vi "lalalala.vi"() -> ()   [LabVIEW 2014]
uses:
  C:/Program Files (x86)/National Instruments/LabVIEW 2014/instr.lib/IDS/ueye.NET/uEyeDotNet.dll
  <vilib>/Analysis/NI_AALBase.lvlib
panel:
  out "Set 2":i32(ring) items=["SUCCESS, Success"=0, "IO_REQUEST_FAILED"=2, "CANT_OPEN_DEVICE"=3, "CANT_CLOSE_DEVICE"=4, "CANT_SETUP_MEMORY"=5, "NO_HWND_FOR_ERROR_REPORT"=6, "ERROR_MESSAGE_NOT_CREATED"=7, "ERROR_STRING_NOT_FOUND"=8, "HOOK_NOT_CREATED"=9, "TIMER_NOT_CREATED"=10, "CANT_OPEN_REGISTRY"=11, "CANT_READ_REGISTRY"=12, "CANT_VALIDATE_BOARD"=13, "CANT_GIVE_BOARD_ACCESS"=14, "NO_IMAGE_MEM_ALLOCATED"=15, "CANT_CLEANUP_MEMORY"=16, "CANT_COMMUNICATE_WITH_DRIVER"=17, "FUNCTION_NOT_SUPPORTED_YET"=18, "OPERATING_SYSTEM_NOT_SUPPORTED"=19, "INVALID_VIDEO_IN"=20, "INVALID_IMG_SIZE"=21, "INVALID_ADDRESS"=22, "INVALID_VIDEO_MODE"=23, "INVALID_AGC_MODE"=24, "INVALID_GAMMA_MODE"=25, "INVALID_SYNC_LEVEL"=26, "INVALID_CBARS_MODE"=27, "INVALID_COLOR_MODE"=28, "INVALID_SCALE_FACTOR"=29, "INVALID_IMAGE_SIZE"=30, "INVALID_IMAGE_POS"=31, "INVALID_CAPTURE_MODE"=32, "INVALID_RISC_PROGRAM"=33, "INVALID_BRIGHTNESS"=34, "INVALID_CONTRAST"=35, "INVALID_SATURATION_U"=36, "INVALID_SATURATION_V"=37, "INVALID_HUE"=38, "INVALID_HOR_FILTER_STEP"=39, "INVALID_VERT_FILTER_STEP"=40, "INVALID_EEPROM_READ_ADDRESS"=41, "INVALID_EEPROM_WRITE_ADDRESS"=42, "INVALID_EEPROM_READ_LENGTH"=43, "INVALID_EEPROM_WRITE_LENGTH"=44, "INVALID_BOARD_INFO_POINTER"=45, "INVALID_DISPLAY_MODE"=46, "INVALID_ERR_REP_MODE"=47, "INVALID_BITS_PIXEL"=48, "INVALID_MEMORY_POINTER"=49, "FILE_WRITE_OPEN_ERROR"=50, "FILE_READ_OPEN_ERROR"=51, "FILE_READ_INVALID_BMP_ID"=52, "FILE_READ_INVALID_BMP_SIZE"=53, "FILE_READ_INVALID_BIT_COUNT"=54, "WRONG_KERNEL_VERSION"=55, "RISC_INVALID_XLENGTH"=60, "RISC_INVALID_YLENGTH"=61, "RISC_EXCEED_IMG_SIZE"=62, "DD_MAIN_FAILED"=70, "DD_PRIMSURFACE_FAILED"=71, "DD_SCRN_SIZE_NOT_SUPPORTED"=72, "DD_CLIPPER_FAILED"=73, "DD_CLIPPER_HWND_FAILED"=74, "DD_CLIPPER_CONNECT_FAILED"=75, "DD_BACKSURFACE_FAILED"=76, "DD_BACKSURFACE_IN_SYSMEM"=77, "DD_MDL_MALLOC_ERR"=78, "DD_MDL_SIZE_ERR"=79, "DD_CLIP_NO_CHANGE"=80, "DD_PRIMMEM_NULL"=81, "DD_BACKMEM_NULL"=82, "DD_BACKOVLMEM_NULL"=83, "DD_OVERLAYSURFACE_FAILED"=84, "DD_OVERLAYSURFACE_IN_SYSMEM"=85, "DD_OVERLAY_NOT_ALLOWED"=86, "DD_OVERLAY_COLKEY_ERR"=87, "DD_OVERLAY_NOT_ENABLED"=88, "DD_GET_DC_ERROR"=89, "DD_DDRAW_DLL_NOT_LOADED"=90, "DD_THREAD_NOT_CREATED"=91, "DD_CANT_GET_CAPS"=92, "DD_NO_OVERLAYSURFACE"=93, "DD_NO_OVERLAYSTRETCH"=94, "DD_CANT_CREATE_OVERLAYSURFACE"=95, "DD_CANT_UPDATE_OVERLAYSURFACE"=96, "DD_INVALID_STRETCH"=97, "EV_INVALID_EVENT_NUMBER"=100, "INVALID_MODE"=101, "CANT_FIND_FALCHOOK, CANT_FIND_HOOK"=102, "CANT_GET_HOOK_PROC_ADDR"=103, "CANT_CHAIN_HOOK_PROC"=104, "CANT_SETUP_WND_PROC"=105, "HWND_NULL"=106, "INVALID_UPDATE_MODE"=107, "NO_ACTIVE_IMG_MEM"=108, "CANT_INIT_EVENT"=109, "FUNC_NOT_AVAIL_IN_OS"=110, "CAMERA_NOT_CONNECTED"=111, "SEQUENCE_LIST_EMPTY"=112, "CANT_ADD_TO_SEQUENCE"=113, "LOW_OF_SEQUENCE_RISC_MEM"=114, "IMGMEM2FREE_USED_IN_SEQ"=115, "IMGMEM_NOT_IN_SEQUENCE_LIST"=116, "SEQUENCE_BUF_ALREADY_LOCKED"=117, "INVALID_DEVICE_ID"=118, "INVALID_BOARD_ID"=119, "ALL_DEVICES_BUSY"=120, "HOOK_BUSY"=121, "TIMED_OUT"=122, "NULL_POINTER"=123, "WRONG_HOOK_VERSION"=124, "InvalidParameter, INVALID_PARAMETER"=125, "NOT_ALLOWED"=126, "OUT_OF_MEMORY"=127, "INVALID_WHILE_LIVE"=128, "ACCESS_VIOLATION"=129, "UNKNOWN_ROP_EFFECT"=130, "INVALID_RENDER_MODE"=131, "INVALID_THREAD_CONTEXT"=132, "NO_HARDWARE_INSTALLED"=133, "INVALID_WATCHDOG_TIME"=134, "INVALID_WATCHDOG_MODE"=135, "INVALID_PASSTHROUGH_IN"=136, "ERROR_SETTING_PASSTHROUGH_IN"=137, "FAILURE_ON_SETTING_WATCHDOG"=138, "NO_USB20"=139, "CAPTURE_RUNNING"=140, "MEMORY_BOARD_ACTIVATED"=141, "MEMORY_BOARD_DEACTIVATED"=142, "NO_MEMORY_BOARD_CONNECTED"=143, "TOO_LESS_MEMORY"=144, "IMAGE_NOT_PRESENT"=145, "MEMORY_MODE_RUNNING"=146, "MEMORYBOARD_DISABLED"=147, "TRIGGER_ACTIVATED"=148, "WRONG_KEY"=150, "CRC_ERROR"=151, "NOT_YET_RELEASED"=152, "NOT_CALIBRATED"=153, "WAITING_FOR_KERNEL"=154, "NOT_SUPPORTED"=155, "TRIGGER_NOT_ACTIVATED"=156, "OPERATION_ABORTED"=157, "BAD_STRUCTURE_SIZE"=158, "INVALID_BUFFER_SIZE"=159, "INVALID_PIXEL_CLOCK"=160, "INVALID_EXPOSURE_TIME"=161, "AUTO_EXPOSURE_RUNNING"=162, "CANNOT_CREATE_BB_SURF"=163, "CANNOT_CREATE_BB_MIX"=164, "BB_OVLMEM_NULL"=165, "CANNOT_CREATE_BB_OVL"=166, "NOT_SUPP_IN_OVL_SURF_MODE"=167, "INVALID_SURFACE"=168, "SURFACE_LOST"=169, "RELEASE_BB_OVL_DC"=170, "BB_TIMER_NOT_CREATED"=171, "BB_OVL_NOT_EN"=172, "ONLY_IN_BB_MODE"=173, "INVALID_COLOR_FORMAT"=174, "INVALID_WB_BINNING_MODE"=175, "INVALID_I2C_DEVICE_ADDRESS"=176, "COULD_NOT_CONVERT"=177, "TRANSFER_ERROR"=178, "PARAMETER_SET_NOT_PRESENT"=179, "INVALID_CAMERA_TYPE"=180, "INVALID_HOST_IP_HIBYTE"=181, "CM_NOT_SUPP_IN_CURR_DISPLAYMODE"=182, "NO_IR_FILTER"=183, "STARTER_FW_UPLOAD_NEEDED"=184, "LIBRARY_NOT_FOUND, DR_LIBRARY_NOT_FOUND"=185, "DR_DEVICE_OUT_OF_MEMORY, DEVICE_OUT_OF_MEMORY"=186, "DR_CANNOT_CREATE_SURFACE, CANNOT_CREATE_SURFACE"=187, "CANNOT_CREATE_VERTEX_BUFFER, DR_CANNOT_CREATE_VERTEX_BUFFER"=188, "CANNOT_CREATE_TEXTURE, DR_CANNOT_CREATE_TEXTURE"=189, "CANNOT_LOCK_OVERLAY_SURFACE, DR_CANNOT_LOCK_OVERLAY_SURFACE"=190, "DR_CANNOT_UNLOCK_OVERLAY_SURFACE, CANNOT_UNLOCK_OVERLAY_SURFACE"=191, "CANNOT_GET_OVERLAY_DC, DR_CANNOT_GET_OVERLAY_DC"=192, "DR_CANNOT_RELEASE_OVERLAY_DC, CANNOT_RELEASE_OVERLAY_DC"=193, "DEVICE_CAPS_INSUFFICIENT, DR_DEVICE_CAPS_INSUFFICIENT"=194, "INCOMPATIBLE_SETTING"=195, "DR_NOT_ALLOWED_WHILE_DC_IS_ACTIVE"=196, "DEVICE_ALREADY_PAIRED"=197, "SUBNETMASK_MISMATCH"=198, "SUBNET_MISMATCH"=199, "INVALID_IP_CONFIGURATION"=200, "DEVICE_NOT_COMPATIBLE"=201, "NETWORK_FRAME_SIZE_INCOMPATIBLE"=202, "NETWORK_CONFIGURATION_INVALID"=203, "ERROR_CPU_IDLE_STATES_CONFIGURATION"=204, "NoSuccess, NO_SUCCESS"=-1]
  out "s32Value":i32
  out "f64Value 2":dbl
  out "f64Value":dbl
  out "Set":i32(ring) items=["SUCCESS, Success"=0, "IO_REQUEST_FAILED"=2, "CANT_OPEN_DEVICE"=3, "CANT_CLOSE_DEVICE"=4, "CANT_SETUP_MEMORY"=5, "NO_HWND_FOR_ERROR_REPORT"=6, "ERROR_MESSAGE_NOT_CREATED"=7, "ERROR_STRING_NOT_FOUND"=8, "HOOK_NOT_CREATED"=9, "TIMER_NOT_CREATED"=10, "CANT_OPEN_REGISTRY"=11, "CANT_READ_REGISTRY"=12, "CANT_VALIDATE_BOARD"=13, "CANT_GIVE_BOARD_ACCESS"=14, "NO_IMAGE_MEM_ALLOCATED"=15, "CANT_CLEANUP_MEMORY"=16, "CANT_COMMUNICATE_WITH_DRIVER"=17, "FUNCTION_NOT_SUPPORTED_YET"=18, "OPERATING_SYSTEM_NOT_SUPPORTED"=19, "INVALID_VIDEO_IN"=20, "INVALID_IMG_SIZE"=21, "INVALID_ADDRESS"=22, "INVALID_VIDEO_MODE"=23, "INVALID_AGC_MODE"=24, "INVALID_GAMMA_MODE"=25, "INVALID_SYNC_LEVEL"=26, "INVALID_CBARS_MODE"=27, "INVALID_COLOR_MODE"=28, "INVALID_SCALE_FACTOR"=29, "INVALID_IMAGE_SIZE"=30, "INVALID_IMAGE_POS"=31, "INVALID_CAPTURE_MODE"=32, "INVALID_RISC_PROGRAM"=33, "INVALID_BRIGHTNESS"=34, "INVALID_CONTRAST"=35, "INVALID_SATURATION_U"=36, "INVALID_SATURATION_V"=37, "INVALID_HUE"=38, "INVALID_HOR_FILTER_STEP"=39, "INVALID_VERT_FILTER_STEP"=40, "INVALID_EEPROM_READ_ADDRESS"=41, "INVALID_EEPROM_WRITE_ADDRESS"=42, "INVALID_EEPROM_READ_LENGTH"=43, "INVALID_EEPROM_WRITE_LENGTH"=44, "INVALID_BOARD_INFO_POINTER"=45, "INVALID_DISPLAY_MODE"=46, "INVALID_ERR_REP_MODE"=47, "INVALID_BITS_PIXEL"=48, "INVALID_MEMORY_POINTER"=49, "FILE_WRITE_OPEN_ERROR"=50, "FILE_READ_OPEN_ERROR"=51, "FILE_READ_INVALID_BMP_ID"=52, "FILE_READ_INVALID_BMP_SIZE"=53, "FILE_READ_INVALID_BIT_COUNT"=54, "WRONG_KERNEL_VERSION"=55, "RISC_INVALID_XLENGTH"=60, "RISC_INVALID_YLENGTH"=61, "RISC_EXCEED_IMG_SIZE"=62, "DD_MAIN_FAILED"=70, "DD_PRIMSURFACE_FAILED"=71, "DD_SCRN_SIZE_NOT_SUPPORTED"=72, "DD_CLIPPER_FAILED"=73, "DD_CLIPPER_HWND_FAILED"=74, "DD_CLIPPER_CONNECT_FAILED"=75, "DD_BACKSURFACE_FAILED"=76, "DD_BACKSURFACE_IN_SYSMEM"=77, "DD_MDL_MALLOC_ERR"=78, "DD_MDL_SIZE_ERR"=79, "DD_CLIP_NO_CHANGE"=80, "DD_PRIMMEM_NULL"=81, "DD_BACKMEM_NULL"=82, "DD_BACKOVLMEM_NULL"=83, "DD_OVERLAYSURFACE_FAILED"=84, "DD_OVERLAYSURFACE_IN_SYSMEM"=85, "DD_OVERLAY_NOT_ALLOWED"=86, "DD_OVERLAY_COLKEY_ERR"=87, "DD_OVERLAY_NOT_ENABLED"=88, "DD_GET_DC_ERROR"=89, "DD_DDRAW_DLL_NOT_LOADED"=90, "DD_THREAD_NOT_CREATED"=91, "DD_CANT_GET_CAPS"=92, "DD_NO_OVERLAYSURFACE"=93, "DD_NO_OVERLAYSTRETCH"=94, "DD_CANT_CREATE_OVERLAYSURFACE"=95, "DD_CANT_UPDATE_OVERLAYSURFACE"=96, "DD_INVALID_STRETCH"=97, "EV_INVALID_EVENT_NUMBER"=100, "INVALID_MODE"=101, "CANT_FIND_FALCHOOK, CANT_FIND_HOOK"=102, "CANT_GET_HOOK_PROC_ADDR"=103, "CANT_CHAIN_HOOK_PROC"=104, "CANT_SETUP_WND_PROC"=105, "HWND_NULL"=106, "INVALID_UPDATE_MODE"=107, "NO_ACTIVE_IMG_MEM"=108, "CANT_INIT_EVENT"=109, "FUNC_NOT_AVAIL_IN_OS"=110, "CAMERA_NOT_CONNECTED"=111, "SEQUENCE_LIST_EMPTY"=112, "CANT_ADD_TO_SEQUENCE"=113, "LOW_OF_SEQUENCE_RISC_MEM"=114, "IMGMEM2FREE_USED_IN_SEQ"=115, "IMGMEM_NOT_IN_SEQUENCE_LIST"=116, "SEQUENCE_BUF_ALREADY_LOCKED"=117, "INVALID_DEVICE_ID"=118, "INVALID_BOARD_ID"=119, "ALL_DEVICES_BUSY"=120, "HOOK_BUSY"=121, "TIMED_OUT"=122, "NULL_POINTER"=123, "WRONG_HOOK_VERSION"=124, "InvalidParameter, INVALID_PARAMETER"=125, "NOT_ALLOWED"=126, "OUT_OF_MEMORY"=127, "INVALID_WHILE_LIVE"=128, "ACCESS_VIOLATION"=129, "UNKNOWN_ROP_EFFECT"=130, "INVALID_RENDER_MODE"=131, "INVALID_THREAD_CONTEXT"=132, "NO_HARDWARE_INSTALLED"=133, "INVALID_WATCHDOG_TIME"=134, "INVALID_WATCHDOG_MODE"=135, "INVALID_PASSTHROUGH_IN"=136, "ERROR_SETTING_PASSTHROUGH_IN"=137, "FAILURE_ON_SETTING_WATCHDOG"=138, "NO_USB20"=139, "CAPTURE_RUNNING"=140, "MEMORY_BOARD_ACTIVATED"=141, "MEMORY_BOARD_DEACTIVATED"=142, "NO_MEMORY_BOARD_CONNECTED"=143, "TOO_LESS_MEMORY"=144, "IMAGE_NOT_PRESENT"=145, "MEMORY_MODE_RUNNING"=146, "MEMORYBOARD_DISABLED"=147, "TRIGGER_ACTIVATED"=148, "WRONG_KEY"=150, "CRC_ERROR"=151, "NOT_YET_RELEASED"=152, "NOT_CALIBRATED"=153, "WAITING_FOR_KERNEL"=154, "NOT_SUPPORTED"=155, "TRIGGER_NOT_ACTIVATED"=156, "OPERATION_ABORTED"=157, "BAD_STRUCTURE_SIZE"=158, "INVALID_BUFFER_SIZE"=159, "INVALID_PIXEL_CLOCK"=160, "INVALID_EXPOSURE_TIME"=161, "AUTO_EXPOSURE_RUNNING"=162, "CANNOT_CREATE_BB_SURF"=163, "CANNOT_CREATE_BB_MIX"=164, "BB_OVLMEM_NULL"=165, "CANNOT_CREATE_BB_OVL"=166, "NOT_SUPP_IN_OVL_SURF_MODE"=167, "INVALID_SURFACE"=168, "SURFACE_LOST"=169, "RELEASE_BB_OVL_DC"=170, "BB_TIMER_NOT_CREATED"=171, "BB_OVL_NOT_EN"=172, "ONLY_IN_BB_MODE"=173, "INVALID_COLOR_FORMAT"=174, "INVALID_WB_BINNING_MODE"=175, "INVALID_I2C_DEVICE_ADDRESS"=176, "COULD_NOT_CONVERT"=177, "TRANSFER_ERROR"=178, "PARAMETER_SET_NOT_PRESENT"=179, "INVALID_CAMERA_TYPE"=180, "INVALID_HOST_IP_HIBYTE"=181, "CM_NOT_SUPP_IN_CURR_DISPLAYMODE"=182, "NO_IR_FILTER"=183, "STARTER_FW_UPLOAD_NEEDED"=184, "LIBRARY_NOT_FOUND, DR_LIBRARY_NOT_FOUND"=185, "DR_DEVICE_OUT_OF_MEMORY, DEVICE_OUT_OF_MEMORY"=186, "DR_CANNOT_CREATE_SURFACE, CANNOT_CREATE_SURFACE"=187, "CANNOT_CREATE_VERTEX_BUFFER, DR_CANNOT_CREATE_VERTEX_BUFFER"=188, "CANNOT_CREATE_TEXTURE, DR_CANNOT_CREATE_TEXTURE"=189, "CANNOT_LOCK_OVERLAY_SURFACE, DR_CANNOT_LOCK_OVERLAY_SURFACE"=190, "DR_CANNOT_UNLOCK_OVERLAY_SURFACE, CANNOT_UNLOCK_OVERLAY_SURFACE"=191, "CANNOT_GET_OVERLAY_DC, DR_CANNOT_GET_OVERLAY_DC"=192, "DR_CANNOT_RELEASE_OVERLAY_DC, CANNOT_RELEASE_OVERLAY_DC"=193, "DEVICE_CAPS_INSUFFICIENT, DR_DEVICE_CAPS_INSUFFICIENT"=194, "INCOMPATIBLE_SETTING"=195, "DR_NOT_ALLOWED_WHILE_DC_IS_ACTIVE"=196, "DEVICE_ALREADY_PAIRED"=197, "SUBNETMASK_MISMATCH"=198, "SUBNET_MISMATCH"=199, "INVALID_IP_CONFIGURATION"=200, "DEVICE_NOT_COMPATIBLE"=201, "NETWORK_FRAME_SIZE_INCOMPATIBLE"=202, "NETWORK_CONFIGURATION_INVALID"=203, "ERROR_CPU_IDLE_STATES_CONFIGURATION"=204, "NoSuccess, NO_SUCCESS"=-1]
  out "x/y":dbl
  out "Histogram Graph":T1(graph)
  out "Image":picture
  out "u8Image":u8[](array[numeric])
  out "CopyToArray":i32(ring) items=["SUCCESS, Success"=0, "IO_REQUEST_FAILED"=2, "CANT_OPEN_DEVICE"=3, "CANT_CLOSE_DEVICE"=4, "CANT_SETUP_MEMORY"=5, "NO_HWND_FOR_ERROR_REPORT"=6, "ERROR_MESSAGE_NOT_CREATED"=7, "ERROR_STRING_NOT_FOUND"=8, "HOOK_NOT_CREATED"=9, "TIMER_NOT_CREATED"=10, "CANT_OPEN_REGISTRY"=11, "CANT_READ_REGISTRY"=12, "CANT_VALIDATE_BOARD"=13, "CANT_GIVE_BOARD_ACCESS"=14, "NO_IMAGE_MEM_ALLOCATED"=15, "CANT_CLEANUP_MEMORY"=16, "CANT_COMMUNICATE_WITH_DRIVER"=17, "FUNCTION_NOT_SUPPORTED_YET"=18, "OPERATING_SYSTEM_NOT_SUPPORTED"=19, "INVALID_VIDEO_IN"=20, "INVALID_IMG_SIZE"=21, "INVALID_ADDRESS"=22, "INVALID_VIDEO_MODE"=23, "INVALID_AGC_MODE"=24, "INVALID_GAMMA_MODE"=25, "INVALID_SYNC_LEVEL"=26, "INVALID_CBARS_MODE"=27, "INVALID_COLOR_MODE"=28, "INVALID_SCALE_FACTOR"=29, "INVALID_IMAGE_SIZE"=30, "INVALID_IMAGE_POS"=31, "INVALID_CAPTURE_MODE"=32, "INVALID_RISC_PROGRAM"=33, "INVALID_BRIGHTNESS"=34, "INVALID_CONTRAST"=35, "INVALID_SATURATION_U"=36, "INVALID_SATURATION_V"=37, "INVALID_HUE"=38, "INVALID_HOR_FILTER_STEP"=39, "INVALID_VERT_FILTER_STEP"=40, "INVALID_EEPROM_READ_ADDRESS"=41, "INVALID_EEPROM_WRITE_ADDRESS"=42, "INVALID_EEPROM_READ_LENGTH"=43, "INVALID_EEPROM_WRITE_LENGTH"=44, "INVALID_BOARD_INFO_POINTER"=45, "INVALID_DISPLAY_MODE"=46, "INVALID_ERR_REP_MODE"=47, "INVALID_BITS_PIXEL"=48, "INVALID_MEMORY_POINTER"=49, "FILE_WRITE_OPEN_ERROR"=50, "FILE_READ_OPEN_ERROR"=51, "FILE_READ_INVALID_BMP_ID"=52, "FILE_READ_INVALID_BMP_SIZE"=53, "FILE_READ_INVALID_BIT_COUNT"=54, "WRONG_KERNEL_VERSION"=55, "RISC_INVALID_XLENGTH"=60, "RISC_INVALID_YLENGTH"=61, "RISC_EXCEED_IMG_SIZE"=62, "DD_MAIN_FAILED"=70, "DD_PRIMSURFACE_FAILED"=71, "DD_SCRN_SIZE_NOT_SUPPORTED"=72, "DD_CLIPPER_FAILED"=73, "DD_CLIPPER_HWND_FAILED"=74, "DD_CLIPPER_CONNECT_FAILED"=75, "DD_BACKSURFACE_FAILED"=76, "DD_BACKSURFACE_IN_SYSMEM"=77, "DD_MDL_MALLOC_ERR"=78, "DD_MDL_SIZE_ERR"=79, "DD_CLIP_NO_CHANGE"=80, "DD_PRIMMEM_NULL"=81, "DD_BACKMEM_NULL"=82, "DD_BACKOVLMEM_NULL"=83, "DD_OVERLAYSURFACE_FAILED"=84, "DD_OVERLAYSURFACE_IN_SYSMEM"=85, "DD_OVERLAY_NOT_ALLOWED"=86, "DD_OVERLAY_COLKEY_ERR"=87, "DD_OVERLAY_NOT_ENABLED"=88, "DD_GET_DC_ERROR"=89, "DD_DDRAW_DLL_NOT_LOADED"=90, "DD_THREAD_NOT_CREATED"=91, "DD_CANT_GET_CAPS"=92, "DD_NO_OVERLAYSURFACE"=93, "DD_NO_OVERLAYSTRETCH"=94, "DD_CANT_CREATE_OVERLAYSURFACE"=95, "DD_CANT_UPDATE_OVERLAYSURFACE"=96, "DD_INVALID_STRETCH"=97, "EV_INVALID_EVENT_NUMBER"=100, "INVALID_MODE"=101, "CANT_FIND_FALCHOOK, CANT_FIND_HOOK"=102, "CANT_GET_HOOK_PROC_ADDR"=103, "CANT_CHAIN_HOOK_PROC"=104, "CANT_SETUP_WND_PROC"=105, "HWND_NULL"=106, "INVALID_UPDATE_MODE"=107, "NO_ACTIVE_IMG_MEM"=108, "CANT_INIT_EVENT"=109, "FUNC_NOT_AVAIL_IN_OS"=110, "CAMERA_NOT_CONNECTED"=111, "SEQUENCE_LIST_EMPTY"=112, "CANT_ADD_TO_SEQUENCE"=113, "LOW_OF_SEQUENCE_RISC_MEM"=114, "IMGMEM2FREE_USED_IN_SEQ"=115, "IMGMEM_NOT_IN_SEQUENCE_LIST"=116, "SEQUENCE_BUF_ALREADY_LOCKED"=117, "INVALID_DEVICE_ID"=118, "INVALID_BOARD_ID"=119, "ALL_DEVICES_BUSY"=120, "HOOK_BUSY"=121, "TIMED_OUT"=122, "NULL_POINTER"=123, "WRONG_HOOK_VERSION"=124, "InvalidParameter, INVALID_PARAMETER"=125, "NOT_ALLOWED"=126, "OUT_OF_MEMORY"=127, "INVALID_WHILE_LIVE"=128, "ACCESS_VIOLATION"=129, "UNKNOWN_ROP_EFFECT"=130, "INVALID_RENDER_MODE"=131, "INVALID_THREAD_CONTEXT"=132, "NO_HARDWARE_INSTALLED"=133, "INVALID_WATCHDOG_TIME"=134, "INVALID_WATCHDOG_MODE"=135, "INVALID_PASSTHROUGH_IN"=136, "ERROR_SETTING_PASSTHROUGH_IN"=137, "FAILURE_ON_SETTING_WATCHDOG"=138, "NO_USB20"=139, "CAPTURE_RUNNING"=140, "MEMORY_BOARD_ACTIVATED"=141, "MEMORY_BOARD_DEACTIVATED"=142, "NO_MEMORY_BOARD_CONNECTED"=143, "TOO_LESS_MEMORY"=144, "IMAGE_NOT_PRESENT"=145, "MEMORY_MODE_RUNNING"=146, "MEMORYBOARD_DISABLED"=147, "TRIGGER_ACTIVATED"=148, "WRONG_KEY"=150, "CRC_ERROR"=151, "NOT_YET_RELEASED"=152, "NOT_CALIBRATED"=153, "WAITING_FOR_KERNEL"=154, "NOT_SUPPORTED"=155, "TRIGGER_NOT_ACTIVATED"=156, "OPERATION_ABORTED"=157, "BAD_STRUCTURE_SIZE"=158, "INVALID_BUFFER_SIZE"=159, "INVALID_PIXEL_CLOCK"=160, "INVALID_EXPOSURE_TIME"=161, "AUTO_EXPOSURE_RUNNING"=162, "CANNOT_CREATE_BB_SURF"=163, "CANNOT_CREATE_BB_MIX"=164, "BB_OVLMEM_NULL"=165, "CANNOT_CREATE_BB_OVL"=166, "NOT_SUPP_IN_OVL_SURF_MODE"=167, "INVALID_SURFACE"=168, "SURFACE_LOST"=169, "RELEASE_BB_OVL_DC"=170, "BB_TIMER_NOT_CREATED"=171, "BB_OVL_NOT_EN"=172, "ONLY_IN_BB_MODE"=173, "INVALID_COLOR_FORMAT"=174, "INVALID_WB_BINNING_MODE"=175, "INVALID_I2C_DEVICE_ADDRESS"=176, "COULD_NOT_CONVERT"=177, "TRANSFER_ERROR"=178, "PARAMETER_SET_NOT_PRESENT"=179, "INVALID_CAMERA_TYPE"=180, "INVALID_HOST_IP_HIBYTE"=181, "CM_NOT_SUPP_IN_CURR_DISPLAYMODE"=182, "NO_IR_FILTER"=183, "STARTER_FW_UPLOAD_NEEDED"=184, "LIBRARY_NOT_FOUND, DR_LIBRARY_NOT_FOUND"=185, "DR_DEVICE_OUT_OF_MEMORY, DEVICE_OUT_OF_MEMORY"=186, "DR_CANNOT_CREATE_SURFACE, CANNOT_CREATE_SURFACE"=187, "CANNOT_CREATE_VERTEX_BUFFER, DR_CANNOT_CREATE_VERTEX_BUFFER"=188, "CANNOT_CREATE_TEXTURE, DR_CANNOT_CREATE_TEXTURE"=189, "CANNOT_LOCK_OVERLAY_SURFACE, DR_CANNOT_LOCK_OVERLAY_SURFACE"=190, "DR_CANNOT_UNLOCK_OVERLAY_SURFACE, CANNOT_UNLOCK_OVERLAY_SURFACE"=191, "CANNOT_GET_OVERLAY_DC, DR_CANNOT_GET_OVERLAY_DC"=192, "DR_CANNOT_RELEASE_OVERLAY_DC, CANNOT_RELEASE_OVERLAY_DC"=193, "DEVICE_CAPS_INSUFFICIENT, DR_DEVICE_CAPS_INSUFFICIENT"=194, "INCOMPATIBLE_SETTING"=195, "DR_NOT_ALLOWED_WHILE_DC_IS_ACTIVE"=196, "DEVICE_ALREADY_PAIRED"=197, "SUBNETMASK_MISMATCH"=198, "SUBNET_MISMATCH"=199, "INVALID_IP_CONFIGURATION"=200, "DEVICE_NOT_COMPATIBLE"=201, "NETWORK_FRAME_SIZE_INCOMPATIBLE"=202, "NETWORK_CONFIGURATION_INVALID"=203, "ERROR_CPU_IDLE_STATES_CONFIGURATION"=204, "NoSuccess, NO_SUCCESS"=-1]
  out "Capture":i32(ring) items=["SUCCESS, Success"=0, "IO_REQUEST_FAILED"=2, "CANT_OPEN_DEVICE"=3, "CANT_CLOSE_DEVICE"=4, "CANT_SETUP_MEMORY"=5, "NO_HWND_FOR_ERROR_REPORT"=6, "ERROR_MESSAGE_NOT_CREATED"=7, "ERROR_STRING_NOT_FOUND"=8, "HOOK_NOT_CREATED"=9, "TIMER_NOT_CREATED"=10, "CANT_OPEN_REGISTRY"=11, "CANT_READ_REGISTRY"=12, "CANT_VALIDATE_BOARD"=13, "CANT_GIVE_BOARD_ACCESS"=14, "NO_IMAGE_MEM_ALLOCATED"=15, "CANT_CLEANUP_MEMORY"=16, "CANT_COMMUNICATE_WITH_DRIVER"=17, "FUNCTION_NOT_SUPPORTED_YET"=18, "OPERATING_SYSTEM_NOT_SUPPORTED"=19, "INVALID_VIDEO_IN"=20, "INVALID_IMG_SIZE"=21, "INVALID_ADDRESS"=22, "INVALID_VIDEO_MODE"=23, "INVALID_AGC_MODE"=24, "INVALID_GAMMA_MODE"=25, "INVALID_SYNC_LEVEL"=26, "INVALID_CBARS_MODE"=27, "INVALID_COLOR_MODE"=28, "INVALID_SCALE_FACTOR"=29, "INVALID_IMAGE_SIZE"=30, "INVALID_IMAGE_POS"=31, "INVALID_CAPTURE_MODE"=32, "INVALID_RISC_PROGRAM"=33, "INVALID_BRIGHTNESS"=34, "INVALID_CONTRAST"=35, "INVALID_SATURATION_U"=36, "INVALID_SATURATION_V"=37, "INVALID_HUE"=38, "INVALID_HOR_FILTER_STEP"=39, "INVALID_VERT_FILTER_STEP"=40, "INVALID_EEPROM_READ_ADDRESS"=41, "INVALID_EEPROM_WRITE_ADDRESS"=42, "INVALID_EEPROM_READ_LENGTH"=43, "INVALID_EEPROM_WRITE_LENGTH"=44, "INVALID_BOARD_INFO_POINTER"=45, "INVALID_DISPLAY_MODE"=46, "INVALID_ERR_REP_MODE"=47, "INVALID_BITS_PIXEL"=48, "INVALID_MEMORY_POINTER"=49, "FILE_WRITE_OPEN_ERROR"=50, "FILE_READ_OPEN_ERROR"=51, "FILE_READ_INVALID_BMP_ID"=52, "FILE_READ_INVALID_BMP_SIZE"=53, "FILE_READ_INVALID_BIT_COUNT"=54, "WRONG_KERNEL_VERSION"=55, "RISC_INVALID_XLENGTH"=60, "RISC_INVALID_YLENGTH"=61, "RISC_EXCEED_IMG_SIZE"=62, "DD_MAIN_FAILED"=70, "DD_PRIMSURFACE_FAILED"=71, "DD_SCRN_SIZE_NOT_SUPPORTED"=72, "DD_CLIPPER_FAILED"=73, "DD_CLIPPER_HWND_FAILED"=74, "DD_CLIPPER_CONNECT_FAILED"=75, "DD_BACKSURFACE_FAILED"=76, "DD_BACKSURFACE_IN_SYSMEM"=77, "DD_MDL_MALLOC_ERR"=78, "DD_MDL_SIZE_ERR"=79, "DD_CLIP_NO_CHANGE"=80, "DD_PRIMMEM_NULL"=81, "DD_BACKMEM_NULL"=82, "DD_BACKOVLMEM_NULL"=83, "DD_OVERLAYSURFACE_FAILED"=84, "DD_OVERLAYSURFACE_IN_SYSMEM"=85, "DD_OVERLAY_NOT_ALLOWED"=86, "DD_OVERLAY_COLKEY_ERR"=87, "DD_OVERLAY_NOT_ENABLED"=88, "DD_GET_DC_ERROR"=89, "DD_DDRAW_DLL_NOT_LOADED"=90, "DD_THREAD_NOT_CREATED"=91, "DD_CANT_GET_CAPS"=92, "DD_NO_OVERLAYSURFACE"=93, "DD_NO_OVERLAYSTRETCH"=94, "DD_CANT_CREATE_OVERLAYSURFACE"=95, "DD_CANT_UPDATE_OVERLAYSURFACE"=96, "DD_INVALID_STRETCH"=97, "EV_INVALID_EVENT_NUMBER"=100, "INVALID_MODE"=101, "CANT_FIND_FALCHOOK, CANT_FIND_HOOK"=102, "CANT_GET_HOOK_PROC_ADDR"=103, "CANT_CHAIN_HOOK_PROC"=104, "CANT_SETUP_WND_PROC"=105, "HWND_NULL"=106, "INVALID_UPDATE_MODE"=107, "NO_ACTIVE_IMG_MEM"=108, "CANT_INIT_EVENT"=109, "FUNC_NOT_AVAIL_IN_OS"=110, "CAMERA_NOT_CONNECTED"=111, "SEQUENCE_LIST_EMPTY"=112, "CANT_ADD_TO_SEQUENCE"=113, "LOW_OF_SEQUENCE_RISC_MEM"=114, "IMGMEM2FREE_USED_IN_SEQ"=115, "IMGMEM_NOT_IN_SEQUENCE_LIST"=116, "SEQUENCE_BUF_ALREADY_LOCKED"=117, "INVALID_DEVICE_ID"=118, "INVALID_BOARD_ID"=119, "ALL_DEVICES_BUSY"=120, "HOOK_BUSY"=121, "TIMED_OUT"=122, "NULL_POINTER"=123, "WRONG_HOOK_VERSION"=124, "InvalidParameter, INVALID_PARAMETER"=125, "NOT_ALLOWED"=126, "OUT_OF_MEMORY"=127, "INVALID_WHILE_LIVE"=128, "ACCESS_VIOLATION"=129, "UNKNOWN_ROP_EFFECT"=130, "INVALID_RENDER_MODE"=131, "INVALID_THREAD_CONTEXT"=132, "NO_HARDWARE_INSTALLED"=133, "INVALID_WATCHDOG_TIME"=134, "INVALID_WATCHDOG_MODE"=135, "INVALID_PASSTHROUGH_IN"=136, "ERROR_SETTING_PASSTHROUGH_IN"=137, "FAILURE_ON_SETTING_WATCHDOG"=138, "NO_USB20"=139, "CAPTURE_RUNNING"=140, "MEMORY_BOARD_ACTIVATED"=141, "MEMORY_BOARD_DEACTIVATED"=142, "NO_MEMORY_BOARD_CONNECTED"=143, "TOO_LESS_MEMORY"=144, "IMAGE_NOT_PRESENT"=145, "MEMORY_MODE_RUNNING"=146, "MEMORYBOARD_DISABLED"=147, "TRIGGER_ACTIVATED"=148, "WRONG_KEY"=150, "CRC_ERROR"=151, "NOT_YET_RELEASED"=152, "NOT_CALIBRATED"=153, "WAITING_FOR_KERNEL"=154, "NOT_SUPPORTED"=155, "TRIGGER_NOT_ACTIVATED"=156, "OPERATION_ABORTED"=157, "BAD_STRUCTURE_SIZE"=158, "INVALID_BUFFER_SIZE"=159, "INVALID_PIXEL_CLOCK"=160, "INVALID_EXPOSURE_TIME"=161, "AUTO_EXPOSURE_RUNNING"=162, "CANNOT_CREATE_BB_SURF"=163, "CANNOT_CREATE_BB_MIX"=164, "BB_OVLMEM_NULL"=165, "CANNOT_CREATE_BB_OVL"=166, "NOT_SUPP_IN_OVL_SURF_MODE"=167, "INVALID_SURFACE"=168, "SURFACE_LOST"=169, "RELEASE_BB_OVL_DC"=170, "BB_TIMER_NOT_CREATED"=171, "BB_OVL_NOT_EN"=172, "ONLY_IN_BB_MODE"=173, "INVALID_COLOR_FORMAT"=174, "INVALID_WB_BINNING_MODE"=175, "INVALID_I2C_DEVICE_ADDRESS"=176, "COULD_NOT_CONVERT"=177, "TRANSFER_ERROR"=178, "PARAMETER_SET_NOT_PRESENT"=179, "INVALID_CAMERA_TYPE"=180, "INVALID_HOST_IP_HIBYTE"=181, "CM_NOT_SUPP_IN_CURR_DISPLAYMODE"=182, "NO_IR_FILTER"=183, "STARTER_FW_UPLOAD_NEEDED"=184, "LIBRARY_NOT_FOUND, DR_LIBRARY_NOT_FOUND"=185, "DR_DEVICE_OUT_OF_MEMORY, DEVICE_OUT_OF_MEMORY"=186, "DR_CANNOT_CREATE_SURFACE, CANNOT_CREATE_SURFACE"=187, "CANNOT_CREATE_VERTEX_BUFFER, DR_CANNOT_CREATE_VERTEX_BUFFER"=188, "CANNOT_CREATE_TEXTURE, DR_CANNOT_CREATE_TEXTURE"=189, "CANNOT_LOCK_OVERLAY_SURFACE, DR_CANNOT_LOCK_OVERLAY_SURFACE"=190, "DR_CANNOT_UNLOCK_OVERLAY_SURFACE, CANNOT_UNLOCK_OVERLAY_SURFACE"=191, "CANNOT_GET_OVERLAY_DC, DR_CANNOT_GET_OVERLAY_DC"=192, "DR_CANNOT_RELEASE_OVERLAY_DC, CANNOT_RELEASE_OVERLAY_DC"=193, "DEVICE_CAPS_INSUFFICIENT, DR_DEVICE_CAPS_INSUFFICIENT"=194, "INCOMPATIBLE_SETTING"=195, "DR_NOT_ALLOWED_WHILE_DC_IS_ACTIVE"=196, "DEVICE_ALREADY_PAIRED"=197, "SUBNETMASK_MISMATCH"=198, "SUBNET_MISMATCH"=199, "INVALID_IP_CONFIGURATION"=200, "DEVICE_NOT_COMPATIBLE"=201, "NETWORK_FRAME_SIZE_INCOMPATIBLE"=202, "NETWORK_CONFIGURATION_INVALID"=203, "ERROR_CPU_IDLE_STATES_CONFIGURATION"=204, "NoSuccess, NO_SUCCESS"=-1]
  out "Bits/Pixel 2":i32=8
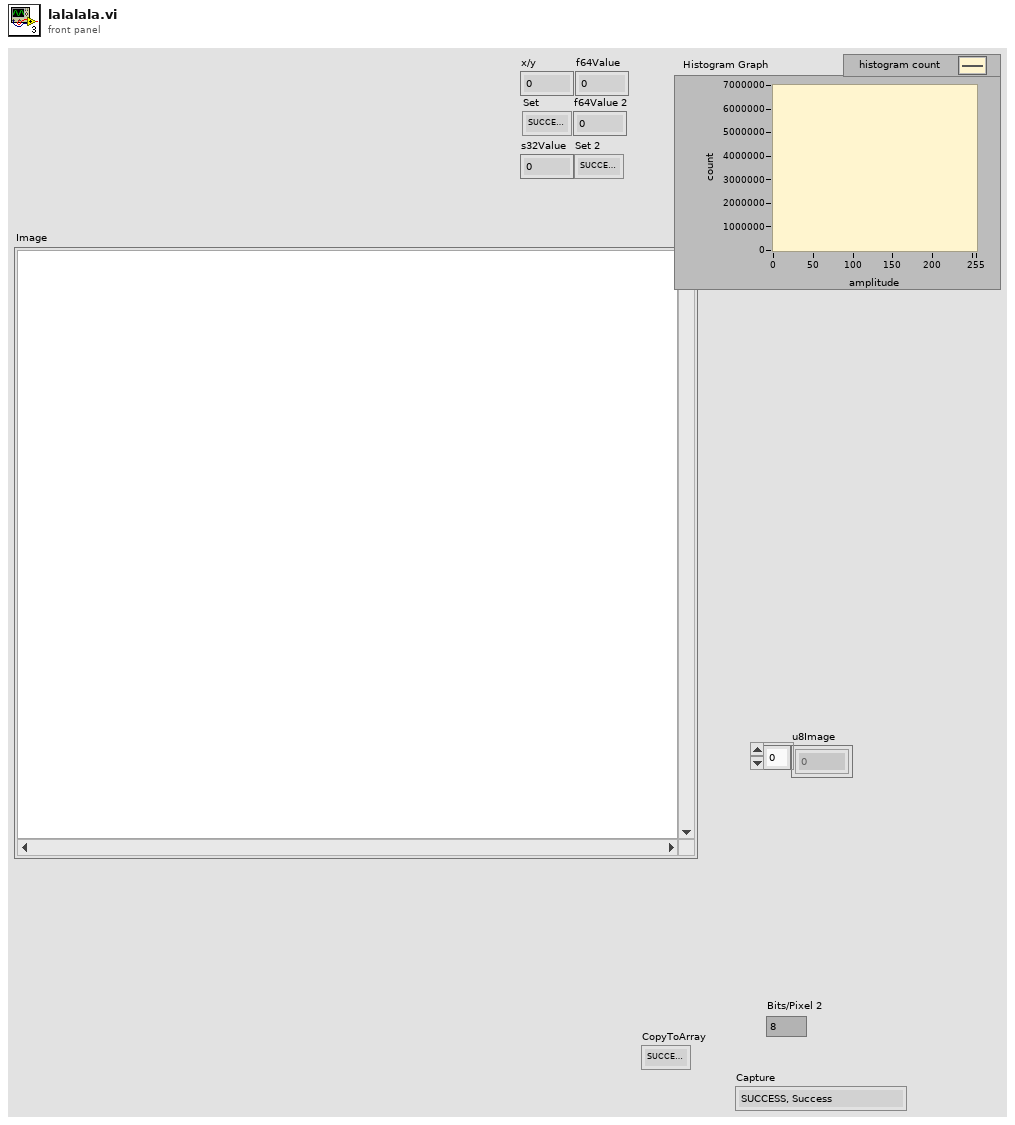
[diagram p1: front panel]
types:
  T1 = cluster{"X Values":dbl[], "Histogram: h(x)":i32[]}
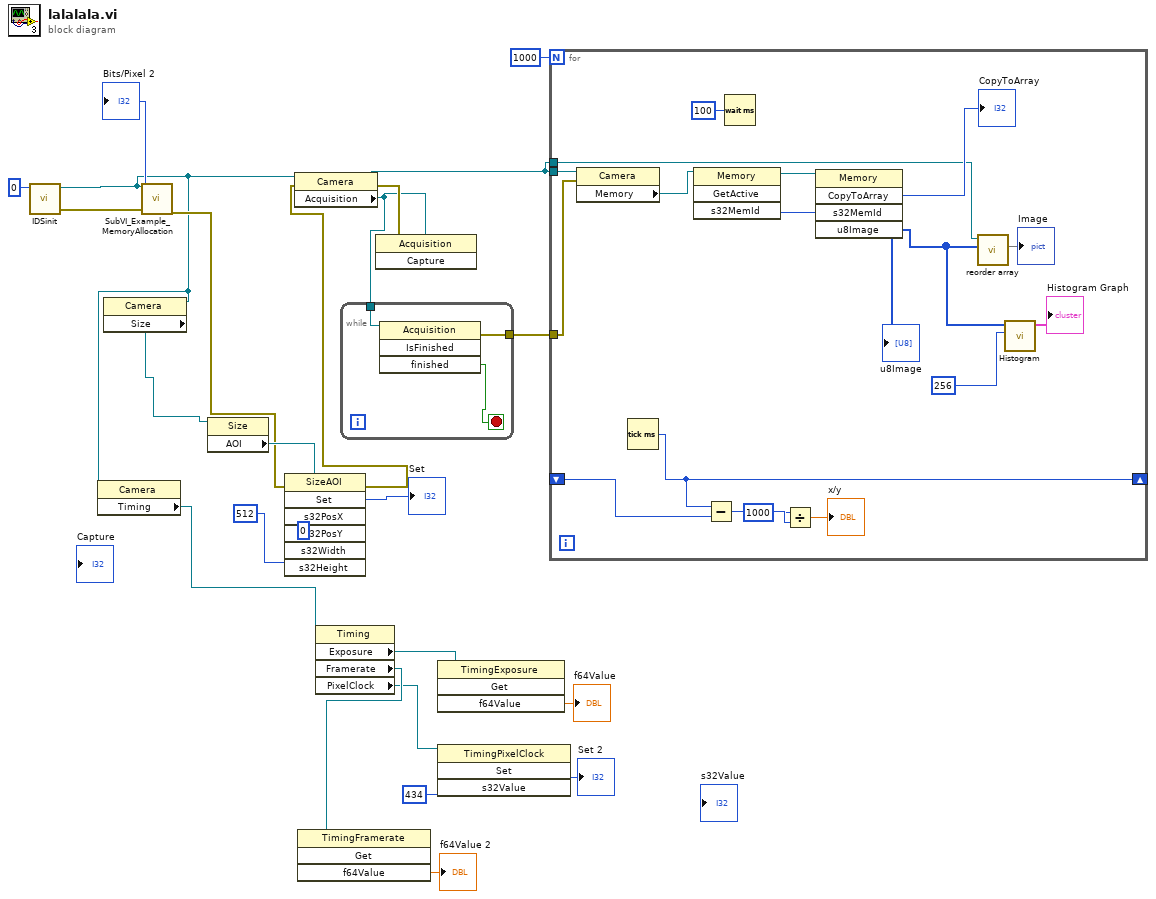
[diagram p0: block diagram]
diagram:
  w10 = 0 ("s32PosY")
  w11 = 512 ("s32PosX")
  n1 = call "IDSinit.vi"("Camera ID"=0) -> ("error out"=w23:errorcluster, "reference out"=w9:refnum<k24>)  [unwired: 7 in, 1 out]
  n2 = property class="Camera"(reference=w9) -> ("Timing"=w8:refnum<k24>)  [unwired: 1 in, 2 out]
  n3 = property class="Camera"(reference=w9) -> ("Size"=w16:refnum<k24>)  [unwired: 1 in, 2 out]
  n4 = call <instrlib>:"SubVI_Example_MemoryAllocation.vi"(".NET (Reference)"=w9, "Error In"=w23) -> ("Bits/Pixel 2"=→"Bits/Pixel 2":i32, "Error Out"=w14:errorcluster)  [unwired: 13 in, 3 out]
  n5 = property class="Size"(reference=w16) -> ("AOI"=w15:refnum<k24>)  [unwired: 1 in, 2 out]
  n6 = invoke class="SizeAOI" method="Set"(reference=w15, error in=w14, "s32PosX"=w10, "s32PosY"=w10, "s32Width"=w11, "s32Height"=w11) -> (error out=w13:errorcluster, "Set"=→"Set":i32)  [unwired: 1 in, 5 out]
  n7 = property class="Camera"(reference=w9, error in=w13) -> (reference out=w20:refnum<k24>, error out=w18:errorcluster, "Acquisition"=w17:refnum<k24>)
  n8 = property class="Timing"(reference=w8) -> ("Exposure"=w7:refnum<k24>, "Framerate"=w5:refnum<k24>, "PixelClock"=w3:refnum<k24>)  [unwired: 1 in, 2 out]
  n9 = invoke class="TimingFramerate" method="Get"(reference=w5) -> ("f64Value"=→"f64Value 2":dbl)  [unwired: 3 in, 3 out]
  n10 = while {
    tunnel: [w27] -> w19
    tunnel: w17 -> [w26]
    stop <- w25 stop-if-true
    n11 = invoke class="Acquisition" method="IsFinished"(reference=w26) -> (error out=w27:errorcluster, "finished"=w25:bool)  [unwired: 3 in, 2 out]
  }
  n12 = invoke class="Acquisition" method="Capture"(reference=w17, error in=w18) -> ()  [unwired: 1 in, 3 out]
  n13 = invoke class="TimingExposure" method="Get"(reference=w7) -> ("f64Value"=→"f64Value":dbl)  [unwired: 3 in, 3 out]
  n14 = invoke class="TimingPixelClock" method="Set"(reference=w3, "s32Value"=434) -> ("Set"=→"Set 2":i32)  [unwired: 2 in, 3 out]
  n15 = for {
    N: 1000 -> [_]
    tunnel: w20 -> [w44]
    tunnel: w20 -> [w38]
    tunnel: w19 -> [w36]
    shift-right: [w32] -> _
    shift-left: _ -> [w31]
    n16 = property class="Camera"(reference=w44, error in=w36) -> ("Memory"=w43:refnum<k24>)  [unwired: 2 out]
    n17 = Tick Count (ms)() -> (millisecond timer value=w32:u32)
    n18 = invoke class="Memory" method="GetActive"(reference=w43) -> (reference out=w42:refnum<k24>, "s32MemId"=w40:i32)  [unwired: 3 in, 2 out]
    n19 = Subtract(x=w32, y=w31) -> (x-y=w30:u32)
    n20 = Wait (ms)(milliseconds to wait=u32 100) -> ()  [unwired: 1 out]
    n21 = Divide(x=u32 1000, y=w30) -> (x/y=→"x/y":dbl)
    n22 = invoke class="Memory" method="CopyToArray"(reference=w42, "s32MemId"=w40) -> ("CopyToArray"=→"CopyToArray":i32, "u8Image"=w35:u8[])  [unwired: 3 in, 3 out]
    "u8Image" <- w35
    n23 = call "reorder array.vi"("InArray"=w35, ".NET (Reference)"=w38) -> (2:→"Image")  [unwired: 7 in, 2 out]
    n24 = call <vilib>:"Histogram.vi"("intervals"=256, "X"=w35) -> ("Histogram Graph"=→"Histogram Graph":T1)  [unwired: 6 in, 3 out]
  }
